vi "SUB_LIST_CurrentFiles.vi"() -> (2 "To Upper Letters":string, 3 "spreadsheet string":string)   [LabVIEW 2011]
panel:
  out "error out":errorcluster
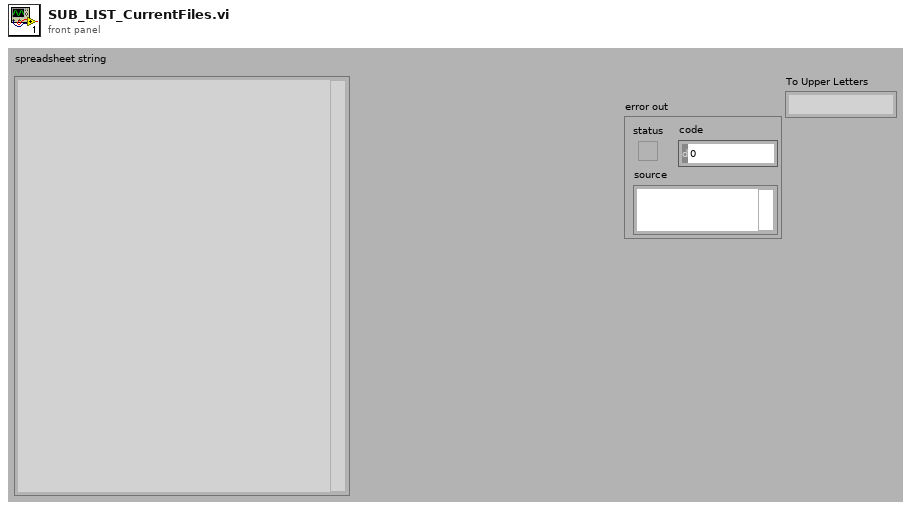
[diagram p1: front panel]
types:
  T1 = enum32{"invalid app kind", "Development System", "Run Time System", "Student Edition", "Embedded LabVIEW", "Evaluation", "Custom"}
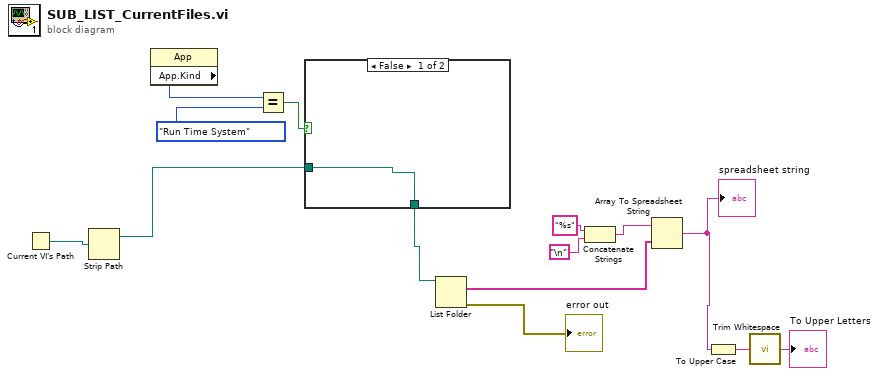
[diagram p0: block diagram]
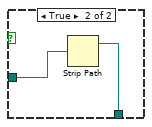
[diagram p2: hidden frame]
diagram:
  n1 = Current VI's Path() -> (path=w14:path)
  n2 = Strip Path(path=w14) -> (stripped path=w10:path)  [unwired: 1 out]
  n3 = property class="App"() -> ("App.Kind"=w11:T1)  [unwired: 2 in, 2 out]
  n4 = Equal?(x=w11, y=T1."Run Time System" ("Application:Kind")) -> (x = y?=w13:bool)
  n5 = case shown="False" w13 {
    tunnel: [w15 w17] -> w9
    tunnel: w10 -> [w15 w16]
    frame False {
    }
    frame True {
      n6 = Strip Path(path=w16) -> (stripped path=w17:path)  [unwired: 1 out]
    }
  }
  n7 = List Folder(path=w9) -> (filenames=w8:string[], error out=→"error out":errorcluster)  [unwired: 3 in, 2 out]
  n8 = Concatenate Strings("%s" ("format string"), "\n") -> (w5:string)
  n9 = Array To Spreadsheet String(array=w8, 3:w5) -> (spreadsheet string=w3:string)  [unwired: 1 in]
  "spreadsheet string" <- w3
  n10 = To Upper Case(1:w3) -> (0:w4:string)
  n11 = call <vilib>:"Trim Whitespace.vi"("string"=w4) -> ("trimmed string"=→"To Upper Letters":string)  [unwired: 1 in]
